vi "Calculate moves.vi"(7 "Position":refnum<class "Position.lvclass">, 8 "error in (no error)":errorcluster, 10 "Source":T1={"File"=enum."d", "Rank"=enum."4"}, 11 "Knight in":refnum<class "Knight.lvclass">) -> (0 "error out":errorcluster, 2 "Moves":refnum<class "Move.lvclass">[](array[class]), 3 "Knight out":refnum<class "Knight.lvclass">)   [LabVIEW 2016, in "Chesslib.lvlib" / "Knight.lvclass"]
uses:
  Knight.lvclass
  Moves/Move/Move.lvclass
  typedef/Square.ctl
  typedef/File.ctl
  typedef/Rank.ctl
  Position/Position.lvclass
  Chesslib.lvlib
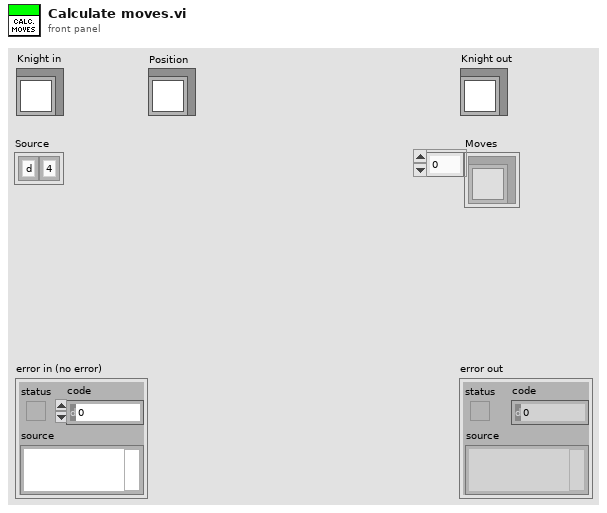
[diagram p1: front panel]
types:
  T1 = typedef "Chesslib.lvlib/Square.ctl" = cluster{"File":T2, "Rank":T3}
  T2 = typedef "Chesslib.lvlib/File.ctl" = enum8{"a", "b", "c", "d", "e", "f", "g", "h"}
  T3 = typedef "Chesslib.lvlib/Rank.ctl" = enum8{"1", "2", "3", "4", "5", "6", "7", "8"}
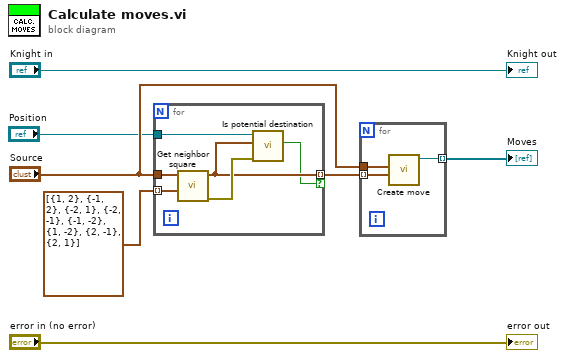
[diagram p0: block diagram]
diagram:
  n1 = for {
    tunnel: "Source" -> [w12]
    tunnel: cluster{i8, i8}[] [{1, 2}, {-1, 2}, {-2, 1}, {-2, -1}, {-1, -2}, {1, -2}, {2, -1}, {2, 1}] -> [w13] mode=indexing
    tunnel: [w10] -> w5 mode=indexing if=w8
    tunnel: "Position" -> [w9]
    n2 = call "Get neighbor square.vi"("Vector (0, 0)"=w13, "Square in"=w12) -> ("error out"=w11:errorcluster, "Square out"=w10:T1)  [unwired: 7 in, 1 out]
    n3 = call "Is potential destination.vi"("error in (no error)"=w11, "Square"=w10, "Position in"=w9) -> ("Potential destination"=w8:bool)  [unwired: 6 in, 2 out]
  }
  n4 = for {
    tunnel: w5 -> [w16] mode=indexing
    tunnel: "Source" -> [w15]
    tunnel: [w14] -> w2 mode=indexing
    n5 = call "Create move.vi"("Destination"=w16, "Source"=w15) -> ("Move out"=w14:refnum<class "Move.lvclass">)  [unwired: 9 in]
  }
  "Moves" <- w2
  "error out" <- "error in (no error)"
  "Knight out" <- "Knight in"
